vi "piezoHoldMidway.vi"() -> ()   [LabVIEW 2017]
panel:
  in  "stop":bool
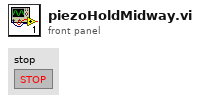
[diagram p1: front panel]
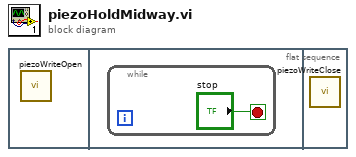
[diagram p0: block diagram]
diagram:
  n1 = flat-sequence {
    frame #0 {
      n2 = call "piezoWriteOpen.vi"() -> ()  [unwired: 2 in]
    }
    frame #1 {
      n3 = while {
        stop <- "stop" stop-if-true
      }
    }
    frame #2 {
      n4 = call "piezoWriteClose.vi"() -> ()  [unwired: 1 in]
    }
  }
